vi "serial to robot.vi"() -> ()   [LabVIEW 2016]
uses:
  E:/Git/projetos Git/SSLView/grSim/grSim Robot Command.ctl
  <vilib>/Instr/_visa.llb/VISA Configure Serial Port (Instr).vi
panel:
  out "string":string
  in  "Robots":T1
  in  "stop":bool
  out "return count":u32
  out "error out":errorcluster
  in  "termination char\n(0xA = '\\n' = LF)":u8=10 format="%.0x"
  in  "VISA resource name":refnum<visa-resource-name>
  in  "Serial Settings":T2={"baud rate"=9600, "data bits"=8, "parity"=enum."None", "stop bits"=10, "flow control"=0} {"flow control" items=["None"=0, "XON/XOFF"=1, "RTS/CTS"=2, "DTR/DSR"=4]; "stop bits" items=["1.0"=10, "1.5"=15, "2.0"=20]; "data bits" min=5 max=8 step=1; "baud rate" items=["75"=75, "110"=110, "134"=134, "150"=150, "300"=300, "600"=600, "1200"=1200, "1800"=1800, "2400"=2400, "4800"=4800, "7200"=7200, "9600"=9600, "14400"=14400, "19200"=19200, "28800"=28800, "38400"=38400, "56000"=56000, "57600"=57600, "115200"=115200, "128000"=128000, "230400"=230400]}
  in  "pos 3":i16=3468
  in  "pos 2":i16=3468
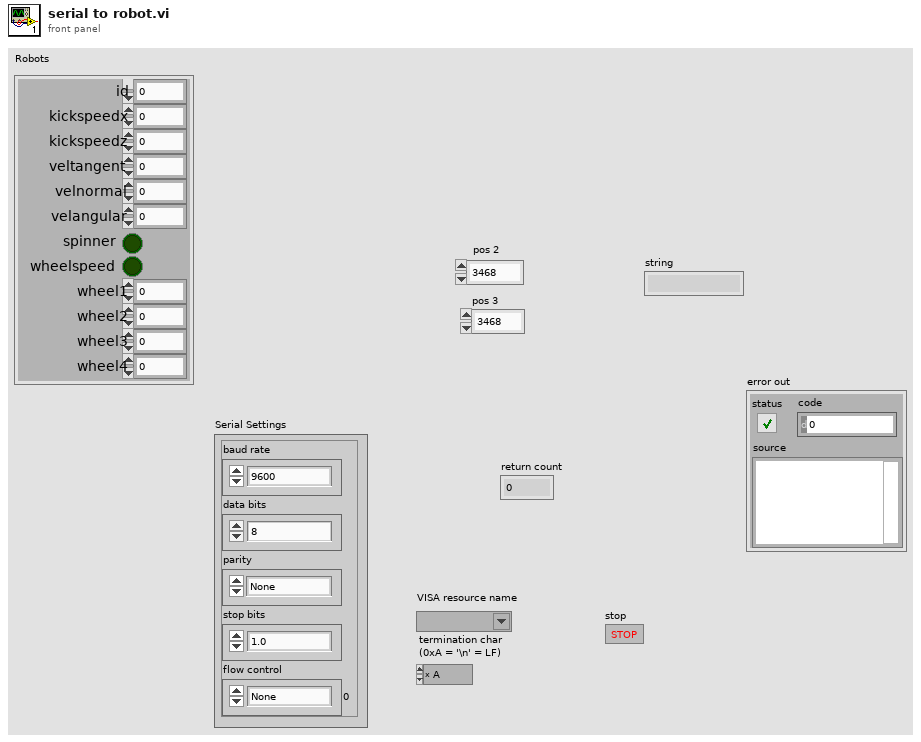
[diagram p1: front panel]
types:
  T1 = typedef "grSim Robot Command.ctl" = cluster{"id":u32, "kickspeedx":sgl, "kickspeedz":sgl, "veltangent":sgl, "velnormal":sgl, "velangular":sgl, "spinner":bool, "wheelspeed":bool, "wheel1":sgl, "wheel2":sgl, "wheel3":sgl, "wheel4":sgl}
  T2 = cluster{"baud rate":u32, "data bits":u16, "parity":enum16{"None", "Odd", "Even", "Mark", "Space"}, "stop bits":u16, "flow control":u16}
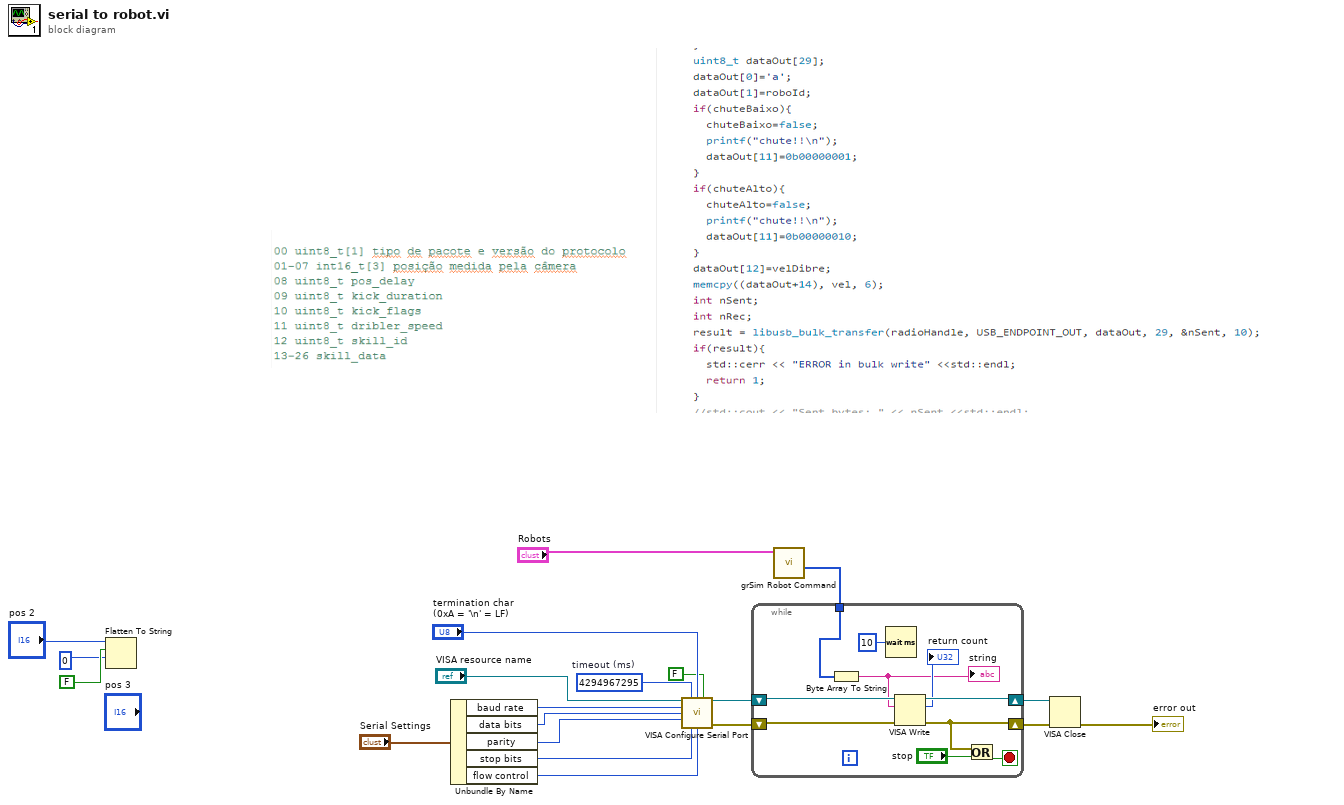
[diagram p0: block diagram]
diagram:
  w3 = u32 4294967295  # timeout (ms)
  n1 = Flatten To String(anything="pos 2", prepend array or string size? (T)=FALSE, byte order (0:big-endian, network order)=u16 0) -> ()  [unwired: 1 in, 3 out]
  n2 = Unbundle By Name("Serial Settings") -> ("baud rate"=w16:u32, "data bits"=w15:u16, "parity"=w14:enum16{"None", "Odd", "Even", "Mark", "Space"}, "stop bits"=w13:u16, "flow control"=w12:u16)
  n3 = call-poly "VISA Configure Serial Port"("VISA resource name"="VISA resource name", "timeout (10sec)"=w3, "termination char\n(0xA = '\\n' = LF)"="termination char\n(0xA = '\\n' = LF)", "Enable Termination\nChar (T)"=FALSE ("Enable Termination\nChar (T)"), "baud rate (9600)"=w16, "data bits (8)"=w15, "parity (0:none)"=w14, "stop bits (10: 1 bit)"=w13, "flow control (0:none)"=w12) -> ("VISA resource name out"=w8:refnum<visa-resource-name>, "error out"=w6:errorcluster)  [unwired: 5 in]
  n4 = call "grSim Robot Command.vi"("Robots"="Robots") -> ("Array"=w2:u8[])  [unwired: 10 in]
  n5 = while {
    shift-right: [w29] -> w7
    shift-left: w8 -> [w30]
    shift-right: [w24] -> w5
    shift-left: w6 -> [w28]
    tunnel: w2 -> [w21]
    stop <- w25 stop-if-true
    n6 = Byte Array To String(unsigned byte array=w21) -> (string=w22:string)
    "string" <- w22
    n7 = Wait (ms)(milliseconds to wait=u32 10) -> ()  [unwired: 1 out]
    n8 = VISA Write(VISA resource name=w30, write buffer=w22, error in (no error)=w28) -> (VISA resource name out=w29:refnum<visa-resource-name>, return count=→"return count":u32, error out=w24:errorcluster)
    n9 = Or(x=w24, y="stop") -> (x .or. y?=w25:bool)
  }
  n10 = VISA Close(VISA resource name=w7, error in (no error)=w5) -> (error out=→"error out":errorcluster)
